vi "Decoder.vi"(0 "Input":string) -> (1 "Registers":T1, 2 "Status Code":string)   [LabVIEW 2010, in "DCP551.lvlib"]
uses:
  DCP551.lvlib
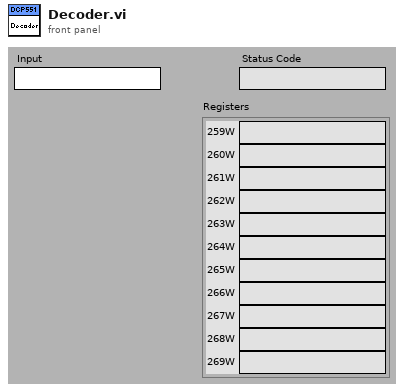
[diagram p1: front panel]
types:
  T1 = cluster{"259W":string, "260W":string, "261W":string, "262W":string, "263W":string, "264W":string, "265W":string, "266W":string, "267W":string, "268W":string, "269W":string}
  T2 = cluster{"[0]":string, "[1]":string, "[2]":string, "[3]":string, "[4]":string, "[5]":string, "[6]":string, "[7]":string, "[8]":string, "[9]":string, "[10]":string}
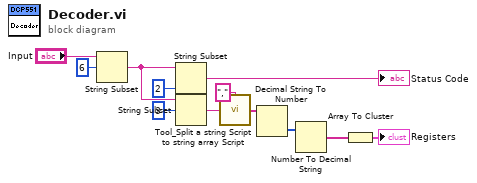
[diagram p0: block diagram]
diagram:
  n1 = String Subset(string="Input", offset (0)=6) -> (substring=w9:string)  [unwired: 1 in]
  n2 = String Subset(string=w9, length (rest)=2 ("offset (0)")) -> (substring=→"Status Code":string)  [unwired: 1 in]
  n3 = String Subset(string=w9, offset (0)=3) -> (substring=w12:string)  [unwired: 1 in]
  n4 = call "Tool_Split a string Script to string array Script.vi"("search string"=",", "input string"=w12) -> ("Array"=w3:string[])  [unwired: 13 in]
  n5 = Decimal String To Number(string=w3) -> (number=w2:i32[])  [unwired: 2 in, 1 out]
  n6 = Number To Decimal String(number=w2) -> (decimal integer string=w1:string[])  [unwired: 1 in]
  n7 = Array To Cluster(array=w1) -> (cluster=→"Registers":T2)
